vi "Close.vi"(8 "error in (no error)":errorcluster, 11 "KNF Settings":T1={"VISA resource name"="", "Simulated?"=TRUE}) -> (0 "error out":errorcluster, 3 "KNF Settings":T1={"VISA resource name"="", "Simulated?"=TRUE})   [LabVIEW 2018, in "KNF SIMDOS.lvlib"]
uses:
  KNF SIMDOS.lvlib
  Settings Cluster plus SIMDOS.ctl
  <vilib>/KNF LAB/Driver S/Lvlib/SIMLAB_driver_lvclass/SIMLAB_driver.lvclass
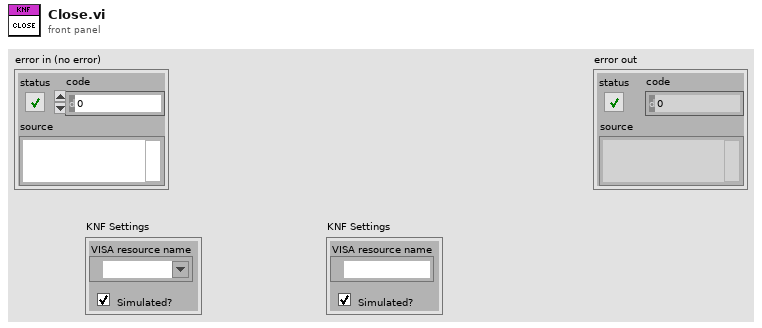
[diagram p1: front panel]
types:
  T1 = typedef "KNF SIMDOS.lvlib/Settings Cluster plus SIMDOS.ctl" = cluster{"VISA resource name":refnum<visa-resource-name>, "Simulated?":bool}
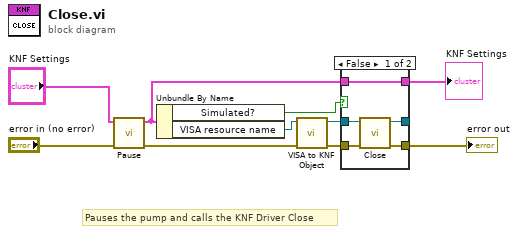
[diagram p0: block diagram]
diagram:
  # "Pauses the pump and calls the KNF Driver Close"
  n1 = call "Pause.vi"("error in (no error)"="error in (no error)", "KNF Settings"="KNF Settings") -> ("error out"=w3:errorcluster, "KNF Settings"=w1:T1)  [unwired: 8 in]
  n2 = Unbundle By Name(w1) -> ("Simulated?"=w10:bool, "VISA resource name"=w8:refnum<visa-resource-name>)
  n3 = call "VISA to KNF Object.vi"("error in (no error)"=w3, "VISA resource name"=w8) -> ("error out"=w6:errorcluster, "SIMDOS out"=w7:refnum<class "SIMLAB_driver.lvclass">)  [unwired: 8 in]
  n4 = case shown="False" w10 {
    tunnel: [w13 w18] -> w5
    tunnel: w1 -> [w13 w18]
    tunnel: [w12 w17] -> w9
    tunnel: w6 -> [w11 w17]
    tunnel: w7 -> [w15 w16]
    tunnel: [w14 w16] -> _
    frame False {
      n5 = call <vilib>:"Close.vi"("error in (no error)"=w11, "SIMDOS in"=w15) -> ("error out"=w12:errorcluster, "SIMDOS out"=w14:refnum<class "SIMLAB_driver.lvclass">)  [unwired: 8 in]
    }
    frame True {
    }
  }
  "error out" <- w9
  "KNF Settings" <- w5
